vi "instantiate_character_splliter.vi"(0 "max_character_length":u32=500, 11 "error in (no error)":errorcluster) -> (4 "chunk_character_splitter out":refnum<class "chunk_character_splitter.lvclass">, 15 "error out":errorcluster)   [LabVIEW 2020, in "chunk_character_splitter.lvclass"]
uses:
  chunk_character_splitter.lvclass
  chunk_character_splitter.lvclass/chunk_character_splitter.ctl
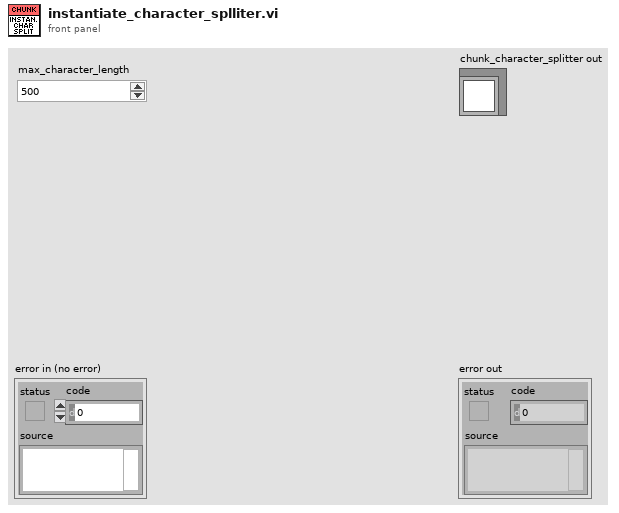
[diagram p1: front panel]
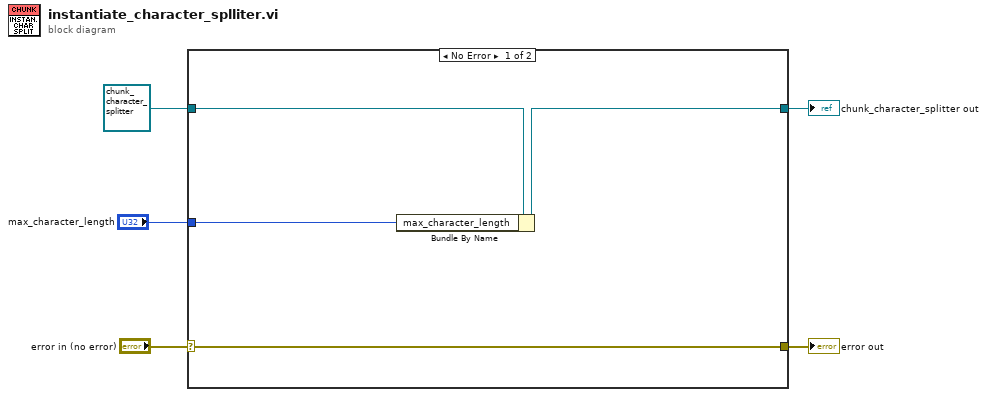
[diagram p0: block diagram]
diagram:
  n1 = case shown="No Error" "error in (no error)" {
    selector: "error in (no error)" -> [w9 w11]
    tunnel: [w9 w11] -> w4
    tunnel: [w6 w10] -> w2
    tunnel: refnum<class "chunk_character_splitter.lvclass"> refnum ("chunk_character_splitter in") -> [w8 w10]
    tunnel: "max_character_length" -> [w7 _]
    frame No Error {
      n2 = Bundle By Name(cluster=w8, "max_character_length"=w7) -> (w6:refnum<class "chunk_character_splitter.lvclass">)
    }
    frame Error {
    }
  }
  "error out" <- w4
  "chunk_character_splitter out" <- w2
